vi "空调型号选择对话框.vi"(11 "枚举":enum16{"黑盾", "英维克"}(ring)) -> (2 "布尔":bool=TRUE, 3 "枚举 2":enum16{"黑盾", "英维克"}(ring))   [LabVIEW 2016, in "环境动力监测库.lvlib" / "空调库.lvlib"]
panel:
  in  "取消":bool
  in  "确定":bool
  # "空调型号选择"
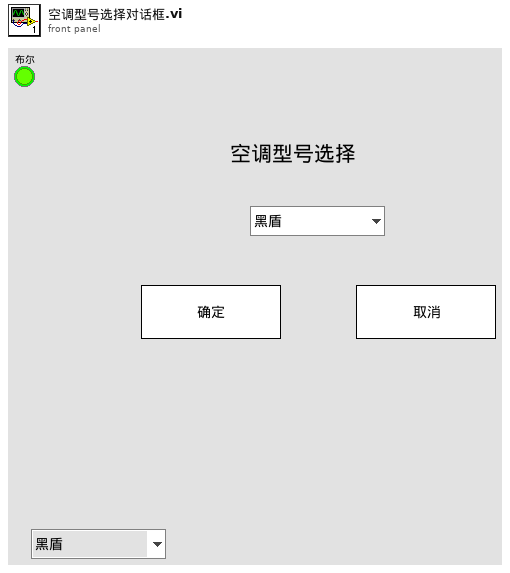
[diagram p1: front panel]
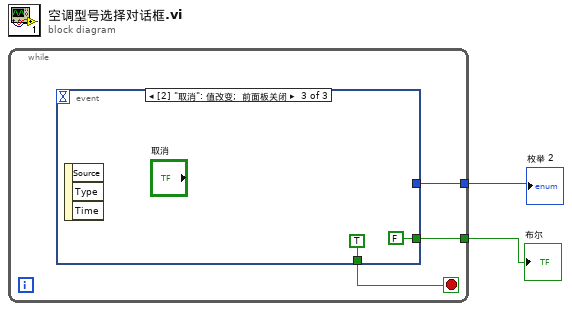
[diagram p0: block diagram]
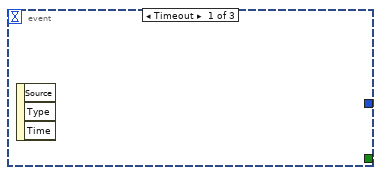
[diagram p2: hidden frame]
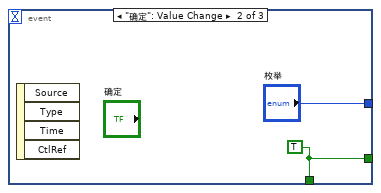
[diagram p3: hidden frame]
diagram:
  n1 = while {
    tunnel: [w5] -> w2
    tunnel: [w3] -> w1
    stop <- w4 stop-if-true
    n2 = event shown="[2] \"取消\": 值改变;  前面板关闭" {
      selector: _ -> [_ _ _]
      dyn-events: _ -> [_ _ _]
      timeout: _ -> [_ _ _]
      tunnel: [_ "枚举" _] -> w5
      tunnel: [_ w6 TRUE] -> w4
      tunnel: [_ w6 FALSE] -> w3
      event Timeout {
        n3 = event-data() -> ()  [unwired: 1 in, 3 out]
      }
      event "确定": Value Change {
        w6 = TRUE
        n4 = event-data() -> ()  [unwired: 1 in, 4 out]
      }
      event "取消": Value Change; Panel Close {
        n5 = event-data() -> ()  [unwired: 1 in, 3 out]
      }
    }
  }
  "枚举 2" <- w2
  "布尔" <- w1
